vi "2D X&Y Commands.vi"(0 "2D wave":string, 1 "minimum":dbl, 2 "maximum":dbl, 5 "X wave":string, 7 "Y wave":string, 9 "X,Y,Z Labels":string[](array[string])=["current (nA)", "field (oe)", "dV/dI (Ohm)"], 11 "error in (no error)":errorcluster, 12 "Kill X&Y waves? [T]":bool=TRUE) -> (4 "result string":string, 15 "error out":errorcluster)   [LabVIEW 2019, in "Data.ITX.lvclass"]
uses:
  Data.ITX.lvclass
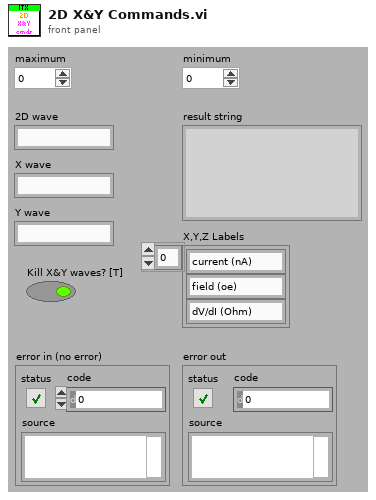
[diagram p1: front panel]
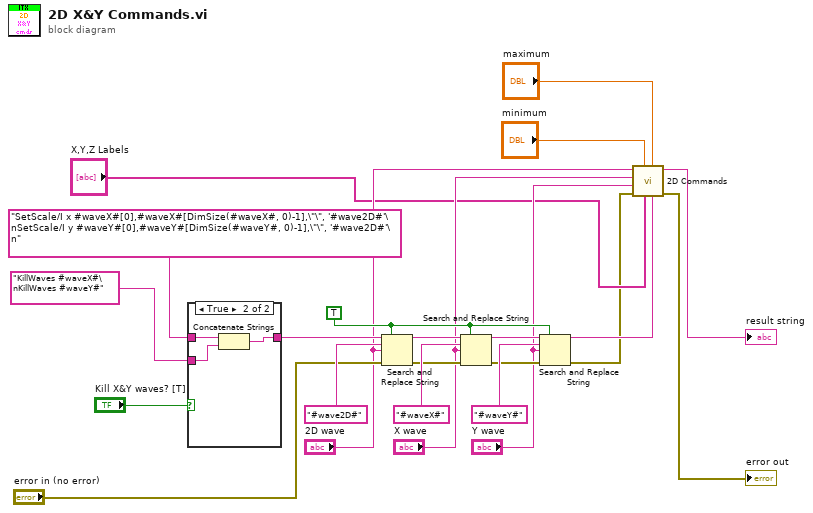
[diagram p0: block diagram]
diagram:
  w23 = TRUE ("replace all? (F)")
  n1 = case shown="True" "Kill X&Y waves? [T]" {
    tunnel: "SetScale/I x #waveX#[0],#waveX#[DimSize(#waveX#, 0)-1],\"\", '#wave2D#'\nSetScale/I y #waveY#[0],#waveY#[DimSize(#waveY#, 0)-1],\"\", '#wave2D#'\n" ("input string 1") -> [w24 w27]
    tunnel: [w24 w26] -> w16
    tunnel: "KillWaves #waveX#\nKillWaves #waveY#" ("input string 2") -> [_ w25]
    frame False {
    }
    frame True {
      n2 = Concatenate Strings(w27, w25) -> (w26:string)
    }
  }
  n3 = Search and Replace String(replace all?=w23, input string=w16, search string="#wave2D#", replace string="2D wave", error in="error in (no error)") -> (result string=w18:string, error out=w12:errorcluster)  [unwired: 5 out]
  n4 = Search and Replace String(replace all?=w23, input string=w18, search string="#waveX#", replace string="X wave", error in=w12) -> (result string=w20:string, error out=w11:errorcluster)  [unwired: 5 out]
  n5 = Search and Replace String(replace all?=w23, input string=w20, search string="#waveY#", replace string="Y wave", error in=w11) -> (result string=w6:string, error out=w4:errorcluster)  [unwired: 5 out]
  n6 = call "2D Commands.vi"("ITX Commands in"=w6, "maximum"="maximum", "X,Y,Z Labels"="X,Y,Z Labels", "minimum"="minimum", "error in (no error)"=w4, "Y wavename"="Y wave", "X wavename"="X wave", "2D wavename"="2D wave") -> ("error out"=→"error out":errorcluster, "result string"=→"result string":string)  [unwired: 2 in]
